vi "Reset_SN.vi"(8 "error in (no error)":errorcluster caption="entrée d'erreur (pas d'erreur)", 11 "Class Creation_SN (Default) en entrée":refnum<class "Creation_SN (Virtual).lvclass">) -> (0 "error out":errorcluster caption="sortie d'erreur", 3 "Class Creation_SN (Default) en sortie":refnum<class "Creation_SN (Virtual).lvclass">)   [LabVIEW 2020, in "Library Instrument & Equipement.lvlib" / "Library Creation_SN.lvlib" / "Creation_SN (Virtual).lvclass"]
uses:
  Creation_SN (Virtual).lvclass
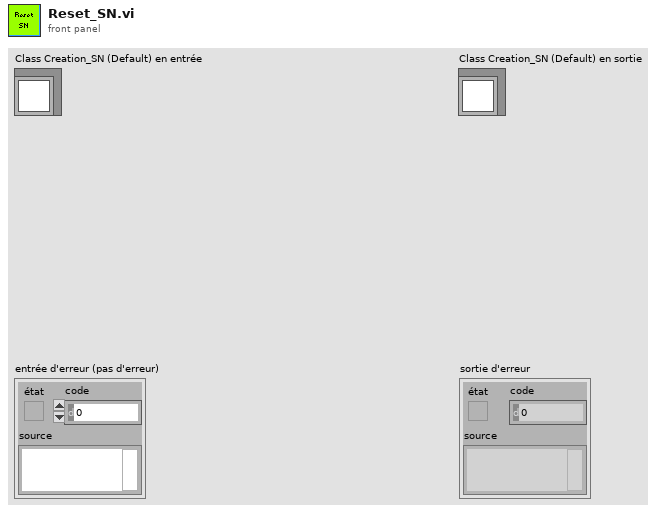
[diagram p1: front panel]
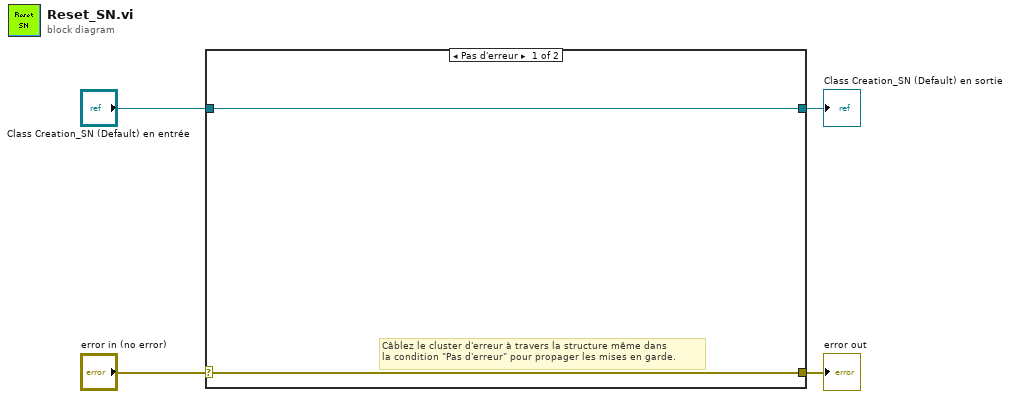
[diagram p0: block diagram]
diagram:
  n1 = case shown="Pas d'erreur" "error in (no error)" {
    selector: "error in (no error)" -> [w5 w8]
    tunnel: [w5 w8] -> w3
    tunnel: [w6 w7] -> w1
    tunnel: "Class Creation_SN (Default) en entrée" -> [w6 w7]
    frame No Error {
      # "Câblez le cluster d'erreur à travers la structure même dans\nla condition \"Pas d'erreur\" pour propager les mises en garde."
    }
    frame Error {
    }
  }
  "error out" <- w3
  "Class Creation_SN (Default) en sortie" <- w1
